vi "Disconnect.vi"(10 "error in (no error)":errorcluster, 11 "Websocket Handler in":refnum<class "Websocket Handler.lvclass">) -> (2 "error out":errorcluster, 3 "Websocket Handler out":refnum<class "Websocket Handler.lvclass">)   [LabVIEW 2020, in "Websocket Handler.lvclass"]
uses:
  <userlib>/lvwamp/Comm Handlers/Websocket Handler/Websocket Handler.lvclass
  <userlib>/lvwamp/Comm Handlers/Websocket Handler/Websocket Handler.lvclass/Websocket Handler.ctl
  <vilib>/MediaMongrels Ltd/WebSockets/WebSockets/WebSocket Client/WebSocket Client.lvclass
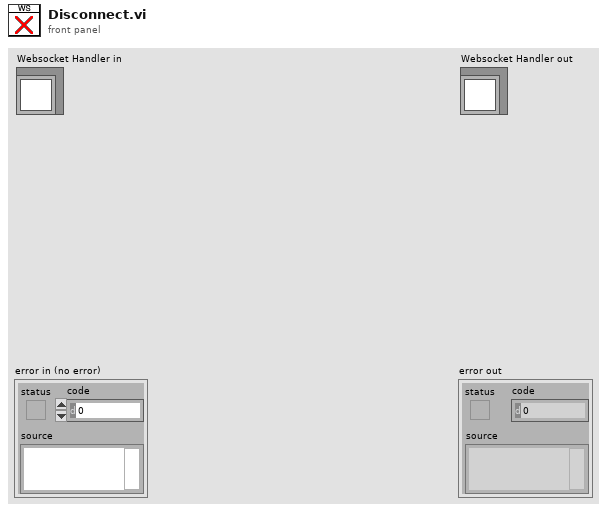
[diagram p1: front panel]
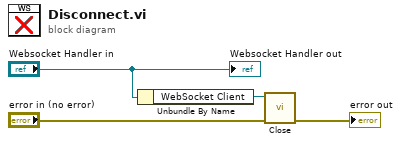
[diagram p0: block diagram]
diagram:
  n1 = Unbundle By Name("Websocket Handler in") -> ("WebSocket Client"=w1:refnum<class "WebSocket Client.lvclass">)
  n2 = call-dynamic "Close.vi"("error in (no error)"="error in (no error)", "WebSocket in"=w1) -> ("error out"=→"error out":errorcluster)  [unwired: 9 in]
  "Websocket Handler out" <- "Websocket Handler in"
